vi "STAV str command.vi"(7 "AddChars":bool, 8 "error in (no error)":errorcluster, 9 "Params":string[](array[string]), 10 "Command":T1) -> (0 "error out":errorcluster, 2 "str command":string)   [LabVIEW 2021, in "STAV lib.lvlib"]
doc: "Use this template to build a VI to use as a subVI."
uses:
  STAV lib.lvlib
  STAV CommandList.ctl
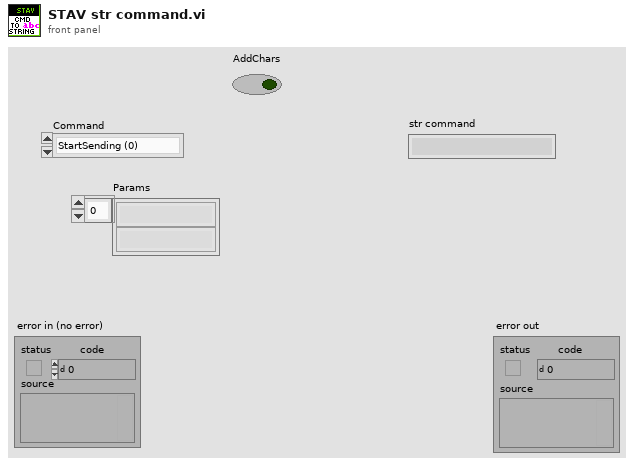
[diagram p1: front panel]
types:
  T1 = typedef "STAV lib.lvlib/STAV CommandList.ctl" = enum16{"StartSending (0)", "StopSending(0)", "FindHomePos(0)", "SetSendingConfig(2)", "GetSendingConfig(0)", "SetPosition(2)", "SetSpeed(2)", "GetSpeed(0)", "GetPosition(0)", "GetForce(0)", "GetPeak(0)", "GetPeakDistance(0)", "GetTravelDistance(0)", "ResetTravelDistance(0)", "GetCycleNo(0)", "GetStepNo(0)", "GetDuration(0)", "GetProfilePosition(0)", "GetHoldTime(0)", "Stop(0)", "StartAndSend(0)", "Start(0)", "Reset(0)", "GetActiveProfile(0)", "SetActiveProfile(2)", "GetProfileCnt(1)", "GetMaxStepCnt(1)", "GetStepCnt(2)", "GetProfileIndex(2)", "SetProfile(3)", "SetStep(3+params)", "GetProfile(2)", "GetStep(3)", "SetProfile(2+params)", ""}
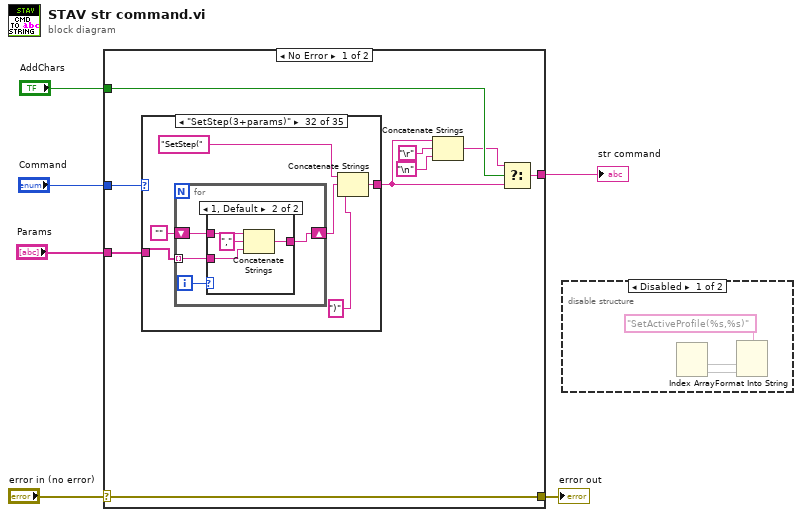
[diagram p0: block diagram]
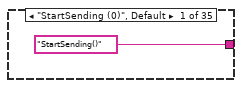
[diagram p3: hidden frame]
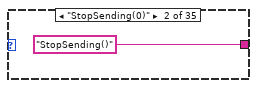
[diagram p4: hidden frame]
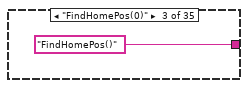
[diagram p5: hidden frame]
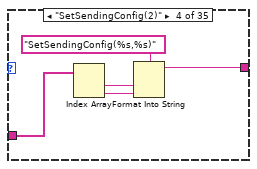
[diagram p6: hidden frame]
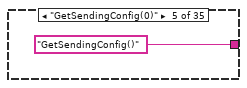
[diagram p7: hidden frame]
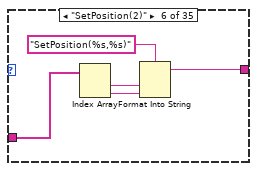
[diagram p8: hidden frame]
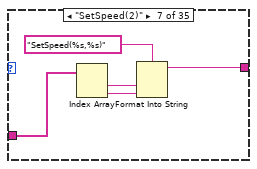
[diagram p9: hidden frame]
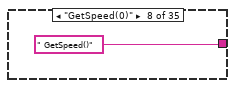
[diagram p10: hidden frame]
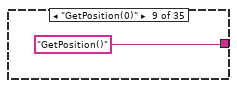
[diagram p11: hidden frame]
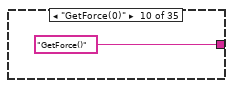
[diagram p12: hidden frame]
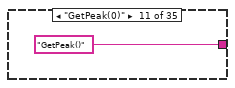
[diagram p13: hidden frame]
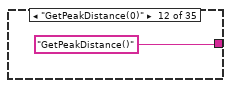
[diagram p14: hidden frame]
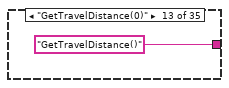
[diagram p15: hidden frame]
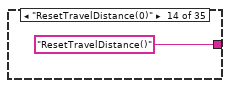
[diagram p16: hidden frame]
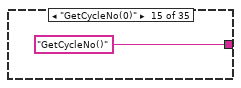
[diagram p17: hidden frame]
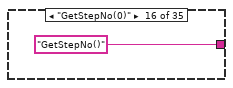
[diagram p18: hidden frame]
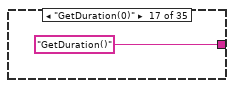
[diagram p19: hidden frame]
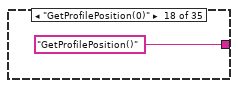
[diagram p20: hidden frame]
diagram:
  n1 = case shown="No Error" "error in (no error)" {
    selector: "error in (no error)" -> [w8 w124]
    tunnel: [w8 w124] -> w5
    tunnel: "Command" -> [w15 _]
    tunnel: "AddChars" -> [w14 _]
    tunnel: [w13 ""] -> w2
    tunnel: "Params" -> [w9 _]
    frame No Error {
      n2 = case shown="\"SetStep(3+params)\"" w15 {
        tunnel: ["StartSending()" "StopSending()" "FindHomePos()" w22 "GetSendingConfig()" w25 w31 " GetSpeed()" "GetPosition()" "GetForce()" "GetPeak()" "GetPeakDistance()" "GetTravelDistance()" "ResetTravelDistance()" "GetCycleNo()" "GetStepNo()" "GetDuration()" "GetProfilePosition()" "GetHoldTime()" "Stop()" "StartAndSend()" "Start()" "Reset()" "GetActiveProfile()" w52 "" w59 w63 w67 w72 w76 w83 w98 w104 w113] -> w7
        tunnel: w9 -> [_ _ _ w21 _ w26 w30 _ _ _ _ _ _ _ _ _ _ _ _ _ _ _ _ _ w53 _ w58 w62 w66 w71 w78 w82 w97 w103 w109]
        frame "StartSending (0)", Default {
        }
        frame "StopSending(0)" {
        }
        frame "FindHomePos(0)" {
        }
        frame "SetSendingConfig(2)" {
          n3 = Index Array(array=w21) -> (element #1=w20:string, element #2=w19:string)  [unwired: 2 in]
          n4 = Format Into String(format string="SetSendingConfig(%s,%s)", w20, w19) -> (resulting string=w22:string)  [unwired: 2 in, 1 out]
        }
        frame "GetSendingConfig(0)" {
        }
        frame "SetPosition(2)" {
          n5 = Index Array(array=w26) -> (element #1=w28:string, element #2=w29:string)  [unwired: 2 in]
          n6 = Format Into String(format string="SetPosition(%s,%s)", w28, w29) -> (resulting string=w25:string)  [unwired: 2 in, 1 out]
        }
        frame "SetSpeed(2)" {
          n7 = Index Array(array=w30) -> (element #1=w33:string, element #2=w34:string)  [unwired: 2 in]
          n8 = Format Into String(format string="SetSpeed(%s,%s)", w33, w34) -> (resulting string=w31:string)  [unwired: 2 in, 1 out]
        }
        frame "GetSpeed(0)" {
        }
        frame "GetPosition(0)" {
        }
        frame "GetForce(0)" {
        }
        frame "GetPeak(0)" {
        }
        frame "GetPeakDistance(0)" {
        }
        frame "GetTravelDistance(0)" {
        }
        frame "ResetTravelDistance(0)" {
        }
        frame "GetCycleNo(0)" {
        }
        frame "GetStepNo(0)" {
        }
        frame "GetDuration(0)" {
        }
        frame "GetProfilePosition(0)" {
        }
        frame "GetHoldTime(0)" {
        }
        frame "Stop(0)" {
        }
        frame "StartAndSend(0)" {
        }
        frame "Start(0)" {
        }
        frame "Reset(0)" {
        }
        frame "GetActiveProfile(0)" {
        }
        frame "SetActiveProfile(2)" {
          n9 = Index Array(array=w53) -> (element #1=w55:string, element #2=w54:string)  [unwired: 2 in]
          n10 = Format Into String(format string="SetActiveProfile(%s,%s)", w55, w54) -> (resulting string=w52:string)  [unwired: 2 in, 1 out]
        }
        frame "" {
        }
        frame "GetProfileCnt(1)" {
          n11 = Index Array(array=w58) -> (element=w60:string)  [unwired: 1 in]
          n12 = Format Into String(format string="GetProfileCnt(%s)", w60) -> (resulting string=w59:string)  [unwired: 2 in, 1 out]
        }
        frame "GetMaxStepCnt(1)" {
          n13 = Index Array(array=w62) -> (element=w64:string)  [unwired: 1 in]
          n14 = Format Into String(format string="GetMaxStepCnt(%s)", w64) -> (resulting string=w63:string)  [unwired: 2 in, 1 out]
        }
        frame "GetStepCnt(2)" {
          n15 = Index Array(array=w66) -> (element #1=w69:string, element #2=w68:string)  [unwired: 2 in]
          n16 = Format Into String(format string="GetStepCnt(%s,%s)", w69, w68) -> (resulting string=w67:string)  [unwired: 2 in, 1 out]
        }
        frame "GetProfileIndex(2)" {
          n17 = Index Array(array=w71) -> (element #1=w74:string, element #2=w73:string)  [unwired: 2 in]
          n18 = Format Into String(format string="GetProfileIndex(%s,%s)", w74, w73) -> (resulting string=w72:string)  [unwired: 2 in, 1 out]
        }
        frame "SetProfile(3)" {
          n19 = Index Array(array=w78) -> (element #1=w80:string, element #2=w79:string, element #3=w77:string)  [unwired: 3 in]
          n20 = Format Into String(format string="SetProfile(%s,%s,%s)", w80, w79, w77) -> (resulting string=w76:string)  [unwired: 2 in, 1 out]
        }
        frame "SetStep(3+params)" {
          n21 = for {
            tunnel: w82 -> [w89] mode=indexing
            shift-right: [w88] -> w87
            shift-left: "" -> [w90]
            i -> [w91]
            n22 = case shown="1, Default" w91 {
              tunnel: w90 -> [_ w96]
              tunnel: w89 -> [w92 w95]
              tunnel: [w92 w93] -> w88
              frame 0 {
              }
              frame 1, Default {
                n23 = Concatenate Strings(w96, "," ("string"), w95) -> (w93:string)
              }
            }
          }
          n24 = Concatenate Strings("SetStep(", w87, ")") -> (w83:string)
        }
        frame "GetProfile(2)" {
          n25 = Index Array(array=w97) -> (element #1=w100:string, element #2=w99:string)  [unwired: 2 in]
          n26 = Format Into String(format string="GetProfile(%s,%s)", w100, w99) -> (resulting string=w98:string)  [unwired: 2 in, 1 out]
        }
        frame "GetStep(3)" {
          n27 = Index Array(array=w103) -> (element #1=w106:string, element #2=w105:string, element #3=w102:string)  [unwired: 3 in]
          n28 = Format Into String(format string="GetStep(%s,%s,%s)", w106, w105, w102) -> (resulting string=w104:string)  [unwired: 2 in, 1 out]
        }
        frame "SetProfile(2+params)" {
          n29 = for {
            tunnel: w109 -> [w115] mode=indexing
            shift-right: [w114] -> w110
            shift-left: "" -> [w116]
            i -> [w117]
            n30 = case shown="1, Default" w117 {
              tunnel: w116 -> [_ w122]
              tunnel: w115 -> [w118 w121]
              tunnel: [w118 w119] -> w114
              frame 0 {
              }
              frame 1, Default {
                n31 = Concatenate Strings(w122, "," ("string"), w121) -> (w119:string)
              }
            }
          }
          n32 = Concatenate Strings("SetProfile(", w110, ")") -> (w113:string)
        }
      }
      n33 = Concatenate Strings(w7, "\r" ("Carriage Return Constant"), "\n" ("Line Feed Constant")) -> (w10:string)
      n34 = Select(t=w10, s=w14, f=w7) -> (s? t:f=w13:string)
    }
    frame Error {
    }
  }
  "error out" <- w5
  "str command" <- w2
  n35 = disable-structure shown="Disabled" {
    frame Disabled {
      n36 = Index Array() -> (array=w128:string[], element #1=w126, element #2=w127)  [unwired: 2 in]
      n37 = Format Into String(format string="SetActiveProfile(%s,%s)", w126, w127) -> ()  [unwired: 2 in, 2 out]
    }
    frame Enabled {
    }
  }
